vi "reflectionPool.vi"(8 "error in (no error)":errorcluster, 9 "action":T2, 10 "object":refnum<class>, 11 "class name":string) -> (0 "error out":errorcluster, 1 "class version numbers":T1(array[cluster]), 2 "class private data":variant[](array[variant]), 3 "class name out":string, 4 "allClassNames":string[](array[string]), 5 "class hierarchy":string[](array[string]))   [LabVIEW 2020, in "JKI JSON Object Serialization.lvlib" / "OOP_Utility.lvlib" / "Reflection.lvclass"]
doc: "GCraftsman JSON Object Serialization Toolkit\nwww.GCraftsman.com\nCopyright (c) 2017, GCraftsman"
uses:
  Reflection.lvclass
  reflectionPoolAction.ctl
  Reflection.lvclass/Reflection.ctl
  determineClassPrivateDataDefaultValue.vi
  determineClassVersion.vi
  <vilib>/Utility/error.llb/Clear Errors.vi
  Get Class Version from Type Descriptor.vi
  <vilib>/Utility/error.llb/Error Cluster From Error Code.vi
  <vilib>/Utility/LVClass/Get LV Class Default Value By Name.vi
  ClassLoader/ClassLoader.lvclass
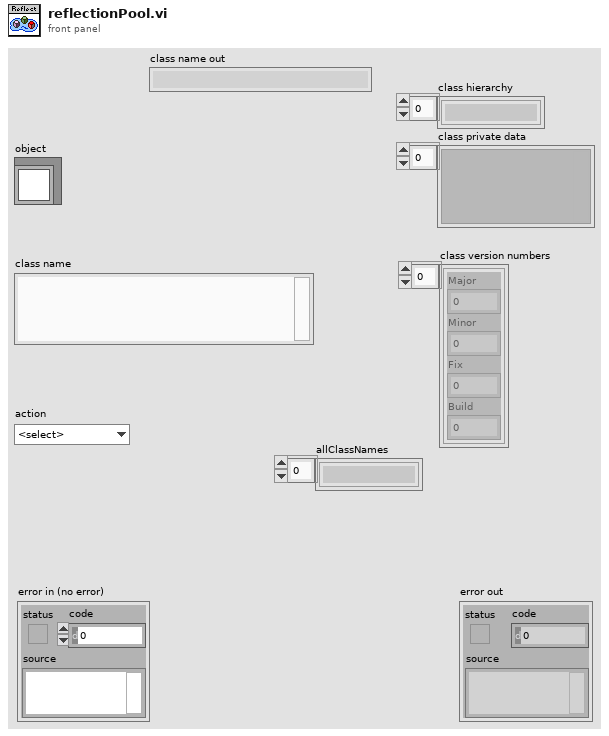
[diagram p1: front panel]
types:
  T1 = cluster{"Major":u16, "Minor":u16, "Fix":u16, "Build":u16}[]
  T2 = typedef "JKI JSON Object Serialization.lvlib/OOP_Utility.lvlib/Reflection.lvclass/reflectionPoolAction.ctl" = enum16{"<select>", "getPrivateData", "getClassHierarchy", "getClassVersions", "getAllClasses"}
  T3 = map{string, cluster{"Major":u16, "Minor":u16, "Fix":u16, "Build":u16}[]}
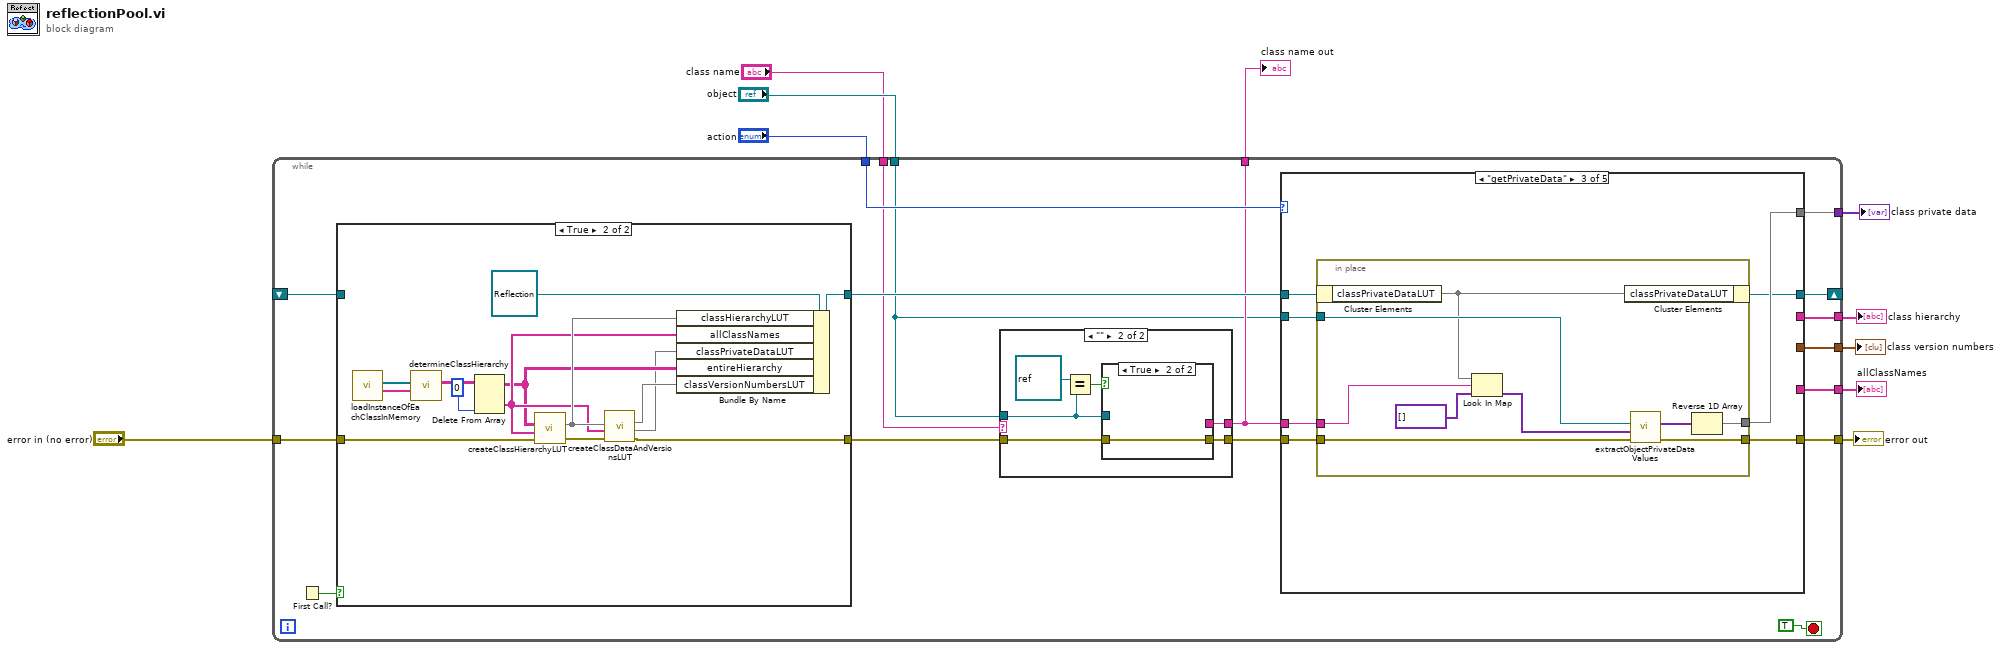
[diagram p0: block diagram]
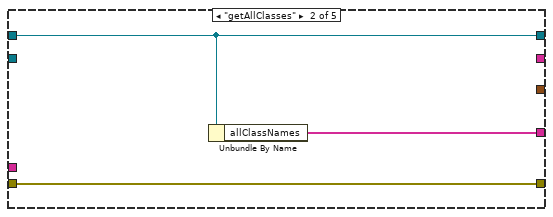
[diagram p3: hidden frame]
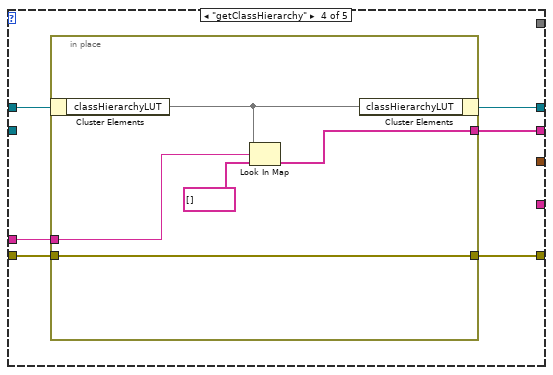
[diagram p4: hidden frame]
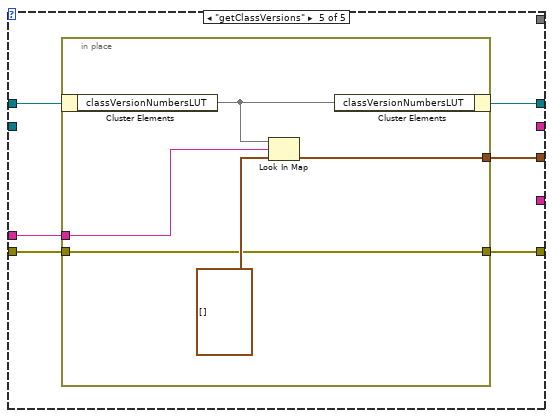
[diagram p5: hidden frame]
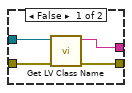
[diagram p7: hidden frame]
diagram:
  n1 = while {
    tunnel: "action" -> [w25]
    shift-right: [w24] -> _
    shift-left: _ -> [w22]
    tunnel: [w21] -> w9
    tunnel: "error in (no error)" -> [w20]
    tunnel: [w19] -> w7
    tunnel: [w18] -> w6
    tunnel: [w17] -> w5
    tunnel: "object" -> [w11]
    tunnel: "class name" -> [w16]
    tunnel: [w13] -> w2
    tunnel: [w12] -> w1
    stop <- TRUE stop-if-true
    n2 = First Call?() -> (First Call?: T/F=w27:bool)
    n3 = case shown="True" w27 {
      tunnel: [w84 w96] -> w15
      tunnel: [w85 w91] -> w23
      tunnel: w22 -> [w85 _]
      tunnel: w20 -> [w84 w87]
      frame False {
      }
      frame True {
        n4 = call "loadInstanceOfEachClassInMemory.vi"() -> ("all class names"=w95:string[], "all classes"=w94:refnum<class>[])  [unwired: 10 in]
        n5 = call "determineClassHierarchy.vi"("classNames"=w95, "classObjects"=w94) -> ("hierarchy"=w98:string[][])  [unwired: 8 in, 1 out]
        n6 = Delete From Array(array=w98, index (col)=0 ("disabled index (col)")) -> (deleted portion=w90:string[], array with subset deleted=w89:string[][])  [unwired: 2 in]
        n7 = call "createClassHierarchyLUT.vi"("error in (no error)"=w87, "allClassNames"=w90, "entireHierarchy"=w89) -> ("error out"=w97:errorcluster, "classHierarchyLUT"=w92:map{string, string[]})  [unwired: 7 in]
        n8 = call "createClassDataAndVersionsLUT.vi"("error in"=w97, "allClassNames"=w90, "classHierarchyLUT"=w92) -> ("error out"=w96:errorcluster, "classPrivateDataLUT"=w86:map{string, variant[]}, "classVersionNumbersLUT"=w88:T3)  [unwired: 5 in, 1 out]
        n9 = Bundle By Name(cluster=refnum<class "Reflection.lvclass"> refnum ("OOP_Utility.lvlib:Reflection.lvclass"), "classHierarchyLUT"=w92, "allClassNames"=w90, "classPrivateDataLUT"=w86, "entireHierarchy"=w89, "classVersionNumbersLUT"=w88) -> (w91:refnum<class "Reflection.lvclass">)
      }
    }
    n10 = case shown="\"\"" w16 {
      selector: w16 -> [w72 _]
      tunnel: [w71 w78] -> w14
      tunnel: w15 -> [w71 w77]
      tunnel: [w72 w76] -> w12
      tunnel: w11 -> [_ w73]
      frame Default {
      }
      frame "" {
        n11 = Equal?(x=refnum<class> refnum ("object"), y=w73) -> (x = y?=w74:bool)
        n12 = case shown="True" w74 {
          tunnel: [w82 w83] -> w78
          tunnel: w77 -> [w81 w83]
          tunnel: [w80 _] -> w76
          tunnel: w73 -> [w79 _]
          frame False {
            n13 = call <vilib>:"Get LV Class Name.vi"("error in (no error)"=w81, "object"=w79) -> ("error out"=w82:errorcluster, "class name"=w80:string)  [unwired: 8 in]
          }
          frame True {
          }
        }
      }
    }
    n14 = case shown="\"getPrivateData\"" w25 {
      tunnel: w14 -> [w29 w32 w35 w53 w65]
      tunnel: [w28 w31 w33 w49 w61] -> w24
      tunnel: w23 -> [w28 w31 w34 w50 w60]
      tunnel: [_ _ w38 _ _] -> w21
      tunnel: [w29 w32 w39 w54 w64] -> w19
      tunnel: [_ _ _ w52 _] -> w18
      tunnel: [_ _ _ _ w63] -> w17
      tunnel: w12 -> [_ _ w37 w51 w62]
      tunnel: w11 -> [_ _ w36 _ _]
      tunnel: [_ w30 _ _ _] -> w13
      frame Default {
      }
      frame "getAllClasses" {
        n15 = Unbundle By Name(w31) -> ("allClassNames"=w30:string[])
      }
      frame "getPrivateData" {
        n16 = in-place {
          in-place-border: [w45] -> w39
          in-place-border: [w44] -> w38
          in-place-border: w37 -> [w43]
          in-place-border: w36 -> [w42]
          in-place-border: w35 -> [w41]
          n17 = in-place-cluster #1(w34) -> ("classPrivateDataLUT"=w40:map{string, variant[]})
          n18 = Look In Map(map=w40, key=w43, default value=variant[] []) -> (value=w46:variant[])  [unwired: 1 out]
          n19 = in-place-cluster #1("classPrivateDataLUT"=w40) -> (w33:refnum<class "Reflection.lvclass">)
          n20 = call "extractObjectPrivateDataValues.vi"("error in (no error)"=w41, "classPrivateDataDefaults"=w46, "Object in"=w42) -> ("error out"=w45:errorcluster, "objectPrivateData"=w48:variant[])  [unwired: 6 in]
          n21 = Reverse 1D Array(array=w48) -> (reversed array=w44:variant[])
        }
      }
      frame "getClassHierarchy" {
        n22 = in-place {
          in-place-border: [w55] -> w54
          in-place-border: w53 -> [w55]
          in-place-border: [w56] -> w52
          in-place-border: w51 -> [w57]
          n23 = in-place-cluster #2(w50) -> ("classHierarchyLUT"=w59:map{string, string[]})
          n24 = Look In Map(map=w59, key=w57, default value=string[] [] ("classNames")) -> (value=w56:string[])  [unwired: 1 out]
          n25 = in-place-cluster #2("classHierarchyLUT"=w59) -> (w49:refnum<class "Reflection.lvclass">)
        }
      }
      frame "getClassVersions" {
        n26 = in-place {
          in-place-border: w65 -> [w67]
          in-place-border: [w67] -> w64
          in-place-border: [w69] -> w63
          in-place-border: w62 -> [w68]
          n27 = in-place-cluster #3(w60) -> ("classVersionNumbersLUT"=w66:T3)
          n28 = Look In Map(map=w66, key=w68, default value=T1 []) -> (value=w69:T1)  [unwired: 1 out]
          n29 = in-place-cluster #3("classVersionNumbersLUT"=w66) -> (w61:refnum<class "Reflection.lvclass">)
        }
      }
    }
  }
  "error out" <- w7
  "class private data" <- w9
  "class hierarchy" <- w6
  "class version numbers" <- w5
  "allClassNames" <- w2
  "class name out" <- w1
